vi "Ballard XML Generator.Open Channel429.vi"(7 "other params":string[](array[string]), 8 "hardware channel":i32, 9 "name":string, 10 "id":string, 11 "string in":string) -> (3 "string out":string)   [LabVIEW 2017]
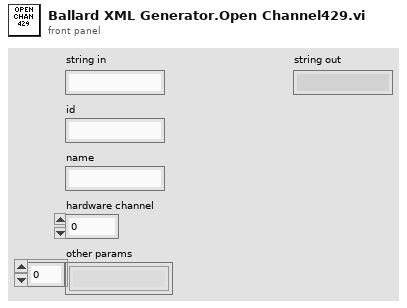
[diagram p1: front panel]
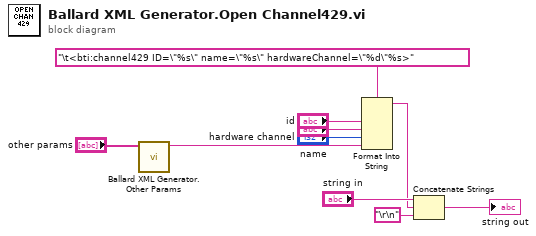
[diagram p0: block diagram]
diagram:
  n1 = call "Ballard XML Generator.Other Params.vi"("other params"="other params") -> ("string"=w1:string)  [unwired: 10 in]
  n2 = Format Into String(format string="\t<bti:channel429 ID=\"%s\" name=\"%s\" hardwareChannel=\"%d\"%s>", "id", "name", "hardware channel", w1) -> (resulting string=w6:string)  [unwired: 2 in, 1 out]
  n3 = Concatenate Strings("string in", w6, "\r\n") -> (→"string out":string)
